vi "DBDTdll.vi"(8 "error in (no error)":errorcluster, 10 "z":dbl[](array[numeric]), 11 "t":dbl) -> (0 "error out":errorcluster, 3 "db out":dbl)   [LabVIEW 2016]
doc: "subroutine DBDT (t,z,db)\n\nCompute the 1st derivative of B (B is the second virial coefficient) with\nrespect to T as a function of temperature and composition.\n\nINPUTS:\n t--temperature [K]\n z--composition [array of mol frac]\n\nOUTPUTS:\n db--1st derivative of B with respect to T [L/mol-K]"
uses:
  REFPROP.DLL
panel:
  # "REFPROP-DBDTdll.vi"
  # "void  DBDTdll(double *t, double *z, double *db)"
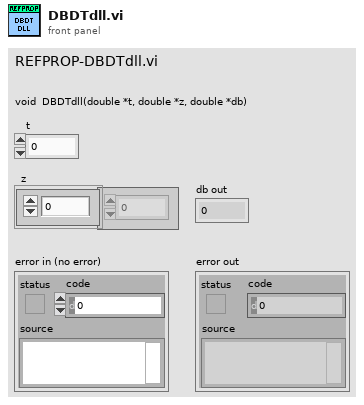
[diagram p1: front panel]
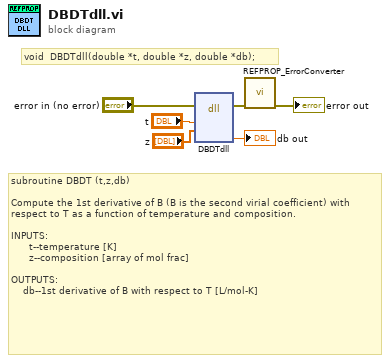
[diagram p0: block diagram]
diagram:
  # "void  DBDTdll(double *t, double *z, double *db);"
  # "subroutine DBDT (t,z,db)\n\nCompute the 1st derivative of B (B is the second virial coefficient) with\nrespect to T as a function of temperature and composition.\n\nINPUTS:\n      t--temperature [K]\n      z--composition [array of mol frac]\n\nOUTPUTS:\n    db--1st derivative of B with respect to T [L/mol-K]"
  n1 = dll-call lib="S:/009 - Testing/02 - Performance Testing/REFPROP/REFPROP.*" fn="DBDTdll"(error in="error in (no error)", "t"="t", "z"="z") -> (error out=w3:errorcluster, "db"=→"db out":dbl)  [unwired: 6 in, 1 out]
  n2 = call "REFPROP_ErrorConverter.vi"("error in (no error)"=w3) -> ("error out"=→"error out":errorcluster)  [unwired: 10 in]
